vi "Set Destination.vi"(8 "error in (no error)":errorcluster, 10 "Destination":refnum<class "DataHandlerAPI.lvclass">, 11 "DataHandlerAPI in":refnum<class "DataHandlerAPI.lvclass">) -> (0 "error out":errorcluster, 3 "DataHandlerAPI out":refnum<class "DataHandlerAPI.lvclass">)   [LabVIEW 2020, in "VolatusData.lvlib" / "DataHandlerAPI.lvclass"]
uses:
  DataHandlerAPI.lvclass
  DataHandlerAPI.lvclass/DataHandlerAPI.ctl
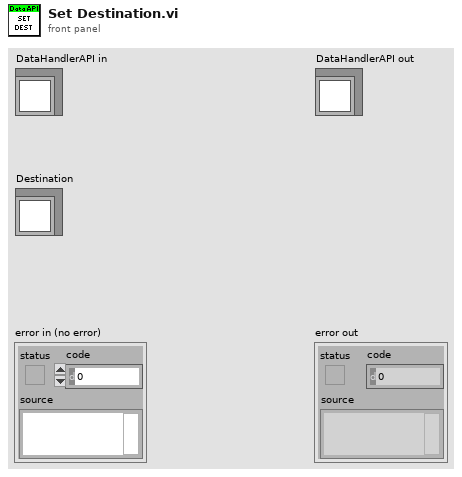
[diagram p1: front panel]
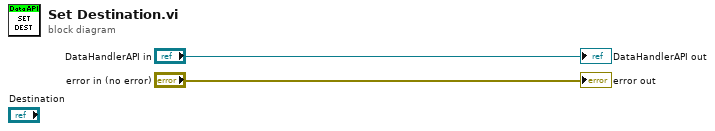
[diagram p0: block diagram]
diagram:
  "error out" <- "error in (no error)"
  "DataHandlerAPI out" <- "DataHandlerAPI in"
